vi "Count_if_Subtrack_Is_Enough_for_Cost_F()-4(2).vi"(3 "[IN] Indexes for Jumps\nfrom Previous Origin":i32[](array[numeric]), 4 "[IN] Index of Problem \nPoint Inside Track":i32, 5 "[IN] Minimal Subtrack Length \n(Points without problems) for\nMaking Desicion":i32, 6 "[IN] Dot Statuses in Track":i16[](array[numeric])) -> (0 "[OUT] Index of Last \nPoint in Track":i32, 2 "[OUT] It's enough to make\nconclusion using subtrack":bool)   [LabVIEW 2017]
doc: "Subprogram calculates how many points before problem point under revision and after (before further problem points) are in the track\n\"101\" points are treated as points without problems..."
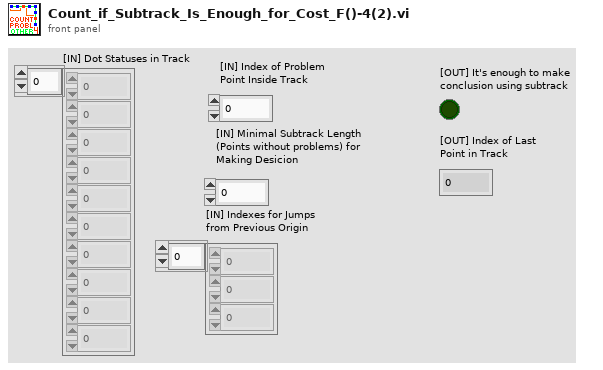
[diagram p1: front panel]
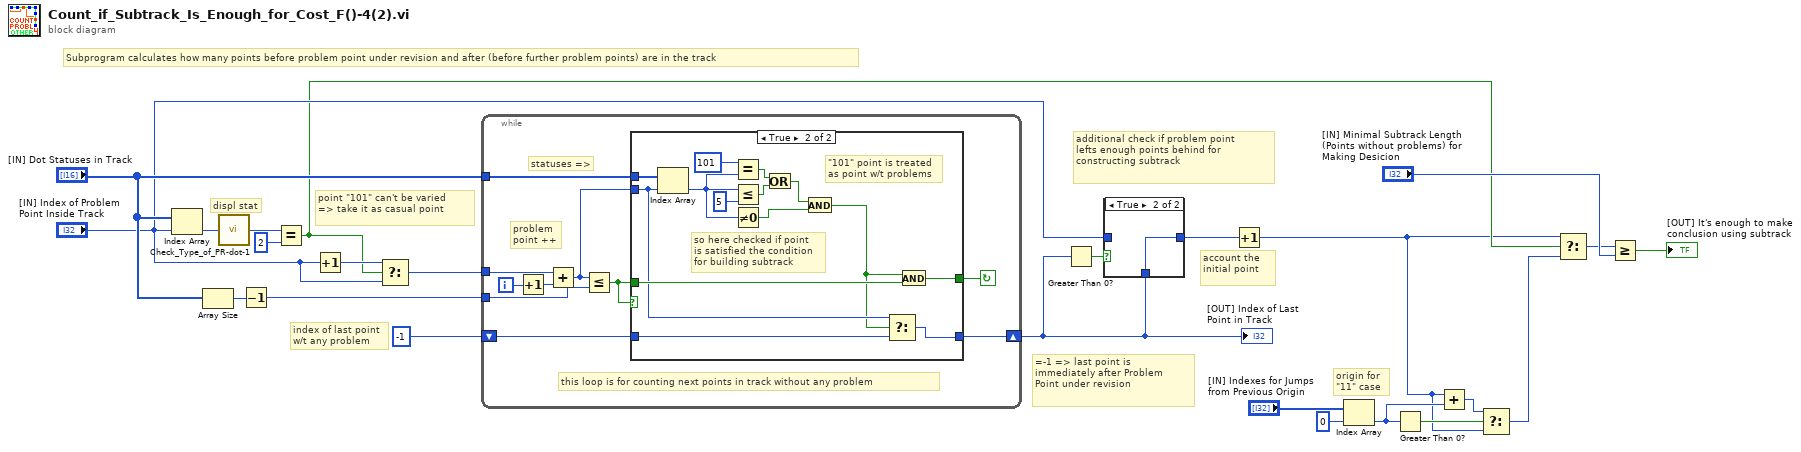
[diagram p0: block diagram]
diagram:
  # "origin for \n\"11\" case"
  # "point \"101\" can't be varied\n=> take it as casual point"
  # "account the \ninitial point"
  # "displ stat"
  # "additional check if problem point \nlefts enough points behind for \nconstructing subtrack"
  # "=-1 => last point is\nimmediately after Problem \nPoint under revision"
  # "Subprogram calculates how many points before problem point under revision and after (before further problem points) are in the track"
  # "index of last point\nw/t any problem"
  n1 = Index Array(array="[IN] Dot Statuses in Track", index="[IN] Index of Problem \nPoint Inside Track") -> (element=w15:i16)
  n2 = Array Size(array="[IN] Dot Statuses in Track") -> (size(s)=w24:i32)
  n3 = call "Check_Type_of_PR-dot-1.vi"("[IN] dot status"=w15) -> ("[OUT] Type of\nproblem dot"=w14:i32)
  n4 = Decrement(x=w24) -> (x-1=w23:i32)
  n5 = Equal?(x=w14, y=2) -> (x = y?=w4:bool)
  n6 = Increment(x="[IN] Index of Problem \nPoint Inside Track") -> (x+1=w12:i32)
  n7 = Select(t=w12, s=w4, f="[IN] Index of Problem \nPoint Inside Track") -> (s? t:f=w10:i32)
  n8 = while {
    tunnel: w23 -> [w32]
    tunnel: w10 -> [w25]
    tunnel: "[IN] Dot Statuses in Track" -> [w31]
    shift-right: [w26] -> w17
    shift-left: -1 -> [w27]
    i -> [w34]
    stop <- w28 continue-if-true
    # "statuses =>"
    # "problem \npoint ++"
    # "this loop is for counting next points in track without any problem"
    n9 = Increment(x=w34) -> (x+1=w33:i32)
    n10 = Add(x=w25, y=w33) -> (x+y=w30:i32)
    n11 = Less Or Equal?(x=w30, y=w32) -> (x <= y?=w29:bool)
    n12 = case shown="True" w29 {
      tunnel: w31 -> [_ w50]
      tunnel: w30 -> [_ w43]
      tunnel: w29 -> [w36 w46]
      tunnel: [w36 w47] -> w28
      tunnel: w27 -> [w35 w44]
      tunnel: [w35 w45] -> w26
      frame False {
        # "it's last point in subtrack"
      }
      frame True {
        # "so here checked if point \nis satisfied the condition \nfor building subtrack"
        # "\"101\" point is treated \nas point w/t problems"
        n13 = Index Array(array=w50, index=w43) -> (element=w41:i16)
        n14 = Equal?(x=i16 101, y=w41) -> (x = y?=w39:bool)
        n15 = Less Or Equal?(x=w41, y=i16 5) -> (x <= y?=w38:bool)
        n16 = Not Equal To 0?(x=w41) -> (x != 0?=w48:bool)
        n17 = Or(x=w39, y=w38) -> (x .or. y?=w37:bool)
        n18 = And(x=w37, y=w48) -> (x .and. y?=w42:bool)
        n19 = Select(t=w43, s=w42, f=w44) -> (s? t:f=w45:i32)
        n20 = And(x=w42, y=w46) -> (x .and. y?=w47:bool)
      }
    }
  }
  "[OUT] Index of Last \nPoint in Track" <- w17
  n21 = Greater Than 0?(x=w17) -> (x > 0?=w19:bool)
  n22 = case shown="True" w19 {
    tunnel: "[IN] Index of Problem \nPoint Inside Track" -> [w51 _]
    tunnel: [w51 w52] -> w18
    tunnel: w17 -> [_ w52]
    frame False {
    }
    frame True {
    }
  }
  n23 = Increment(x=w18) -> (x+1=w3:i32)
  n24 = Index Array(array="[IN] Indexes for Jumps\nfrom Previous Origin", index=0) -> (element=w7:i32)
  n25 = Greater Than 0?(x=w7) -> (x > 0?=w8:bool)
  n26 = Add(x=w3, y=w7) -> (x+y=w6:i32)
  n27 = Select(t=w6, s=w8, f=w3) -> (s? t:f=w1:i32)
  n28 = Select(t=w3, s=w4, f=w1) -> (s? t:f=w2:i32)
  n29 = Greater Or Equal?(x=w2, y="[IN] Minimal Subtrack Length \n(Points without problems) for\nMaking Desicion") -> (x >= y?=→"[OUT] It's enough to make\nconclusion using subtrack":bool)
